vi "Add Linked List to Parent.vi"(4 "Insertion Index":i32=-1, 6 "Linked List ID":string, 7 "Parent ID":string, 8 "error in (no error)":errorcluster, 11 "Linked List in":refnum<class "Linked List.lvclass">) -> (0 "error out":errorcluster, 3 "Linked List out":refnum<class "Linked List.lvclass">)   [LabVIEW 2019, in "Linked Lists.lvlib" / "Linked List.lvclass"]
uses:
  <vilib>/gpm_packages/@cs/linked-list/Source/Linked List/Linked List/Linked List.lvclass
  <vilib>/gpm_packages/@cs/linked-list/Source/Linked List/Linked List Definition/Linked List Definition.lvclass
  <vilib>/gpm_packages/@cs/linked-list/Source/Linked List/Linked List/Linked List.lvclass/Linked List.ctl
  <vilib>/gpm_packages/@cs/lookup-table/Source/LookupTable/LookupTable.lvclass/LookupTable.ctl
  ee1731ca-b18a-4210-8762-6faa4a5b3069.vi
  <vilib>/gpm_packages/@cs/lookup-table/Source/LookupTable/Read Table Reference.vi
  ee1731ca-b18a-4210-8762-6faa4a5b3069.vi/d37d61dc-18a1-4215-aeae-0f6cc9253f1b.vi
  <vilib>/gpm_packages/@cs/lookup-table/Source/LookupTable/LookupTable.lvclass
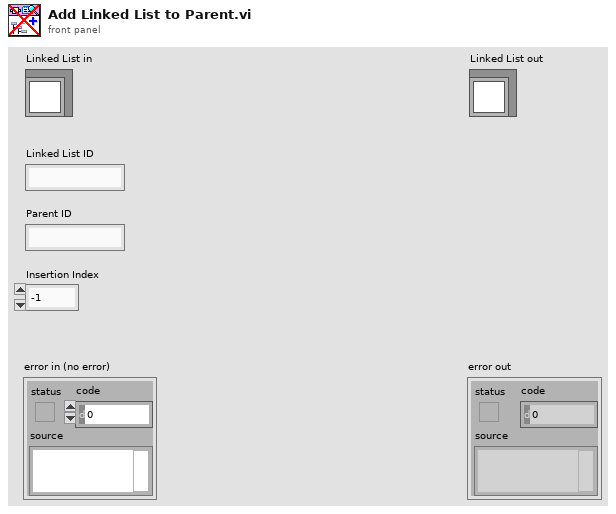
[diagram p1: front panel]
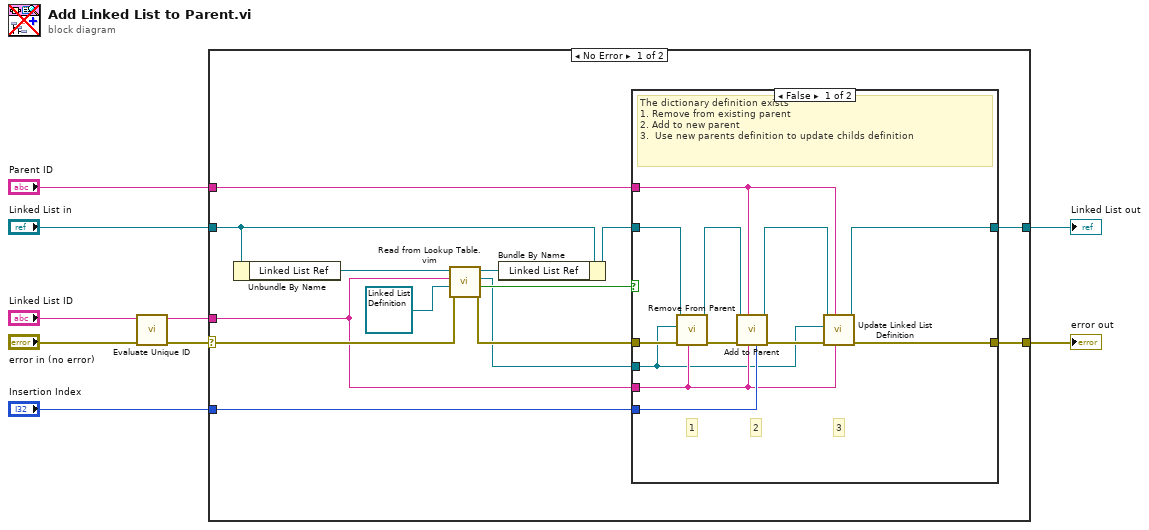
[diagram p0: block diagram]
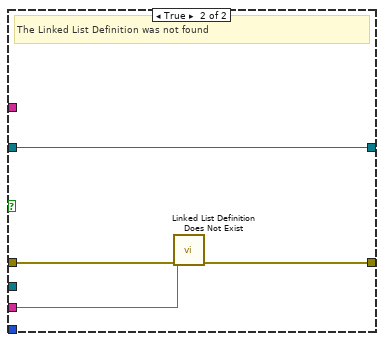
[diagram p2: hidden frame]
diagram:
  n1 = call <vilib>:"Evaluate Unique ID.vi"("error in (no error)"="error in (no error)", "Unique ID"="Linked List ID") -> ("error out"=w7:errorcluster, "Unique ID Out"=w4:string)  [unwired: 8 in]
  n2 = case shown="No Error" w7 {
    selector: w7 -> [w21 w40]
    tunnel: [w17 w41] -> w5
    tunnel: "Linked List in" -> [w15 w41]
    tunnel: w4 -> [w12 _]
    tunnel: [w18 w40] -> w3
    tunnel: "Insertion Index" -> [w11 _]
    tunnel: "Parent ID" -> [w10 _]
    frame No Error {
      n3 = Unbundle By Name(w15) -> ("Linked List Ref"=w23:refnum<data-value>)
      n4 = call "Read from Lookup Table.vim"("error in (no error)"=w21, "Type"=refnum<class "Linked List Definition.lvclass"> refnum ("Linked List.lvlib:Linked List Definition.lvclass"), "Item Name"=w12, "LookupTable Reference"=w23) -> ("error out"=w19:errorcluster, "Not Found?"=w20:bool, "Value"=w13:refnum<class "Linked List Definition.lvclass">, "LookupTable Reference Out"=w16:refnum<data-value>)  [unwired: 4 in]
      n5 = Bundle By Name(cluster=w15, "Linked List Ref"=w16) -> (w14:refnum<class "Linked List.lvclass">)
      n6 = case shown="False" w20 {
        tunnel: [w29 w37] -> w18
        tunnel: w19 -> [w34 w38]
        tunnel: [w27 w39] -> w17
        tunnel: w14 -> [w35 w39]
        tunnel: w13 -> [w24 _]
        tunnel: w12 -> [w25 w36]
        tunnel: w11 -> [w31 _]
        tunnel: w10 -> [w26 _]
        frame False {
          # "3"
          # "2"
          # "1"
          # "The dictionary definition exists\n1. Remove from existing parent\n2. Add to new parent\n3.  Use new parents definition to update childs definition"
          n7 = call <vilib>:"Remove From Parent.vi"("Unique ID"=w25, "error in (no error)"=w34, "Linked List Definition"=w24, "Linked List in"=w35) -> ("error out"=w32:errorcluster, "Linked List out"=w33:refnum<class "Linked List.lvclass">)  [unwired: 6 in]
          n8 = call <vilib>:"Add to Parent.vi"("Insertion Index"=w31, "Unique ID"=w25, "Parent ID"=w26, "error in (no error)"=w32, "Linked List in"=w33) -> ("error out"=w30:errorcluster, "Linked List out"=w28:refnum<class "Linked List.lvclass">)  [unwired: 5 in]
          n9 = call <vilib>:"Update Linked List Definition.vi"("Unique ID"=w25, "Parent ID"=w26, "error in (no error)"=w30, "Linked List Definition"=w24, "Linked List in"=w28) -> ("error out"=w29:errorcluster, "Linked List out"=w27:refnum<class "Linked List.lvclass">)  [unwired: 5 in]
        }
        frame True {
          # "The Linked List Definition was not found"
          n10 = call <vilib>:"Linked List Definition Does Not Exist.vi"("Error In"=w38, "Unique ID"=w36) -> ("Error Out"=w37:errorcluster)  [unwired: 9 in]
        }
      }
    }
    frame Error {
    }
  }
  "error out" <- w3
  "Linked List out" <- w5
